vi "DimostratoreCalibrazioni-backup.vi"() -> ()   [LabVIEW 2019]
uses:
  TypeDef/SlugExpiration.ctl
  ByteGSAPIBase.lvclass
  TypeDef/CalibrationStates.ctl
  FetchCalibration/Converted_Slug_Cluster.ctl
  Instruments/Instruments.ctl
  CalibrationMeasurements/BodyCalibrazioneMisure.ctl
  aa47c742-c095-4670-bf1f-6b28e4309cef.vi
  <vilib>/numeric/Random Number (Range) I64.vi
  <vilib>/Array/Sort 2D Array - Pop Stack.vi
  <vilib>/Array/Sort 2D Array - Push Stack.vi
  <vilib>/numeric/sub_Random U32.vi
panel:
  out "Stato":string
  out "Misurazioni n.":string
  in  "Cancel":bool
  in  "Approvation":bool
  out "Tot Misurazioni":i32
  in  "Avanti":bool
  in  "Repeat":bool
  out "Esito":string
  out "Valore misurato":dbl
  out "Valore di riferimento":dbl
  out "Waveform Chart":i64(graph)
  in  "Start Calibration":bool
  in  "Next":bool
  in  "Previus":bool
  out "Misurazioni":string
  in  "Filtro":enum16{"All", "Expired", "Not Expired"}(ring)
  in  "Slug list":T1[](array[typedef])
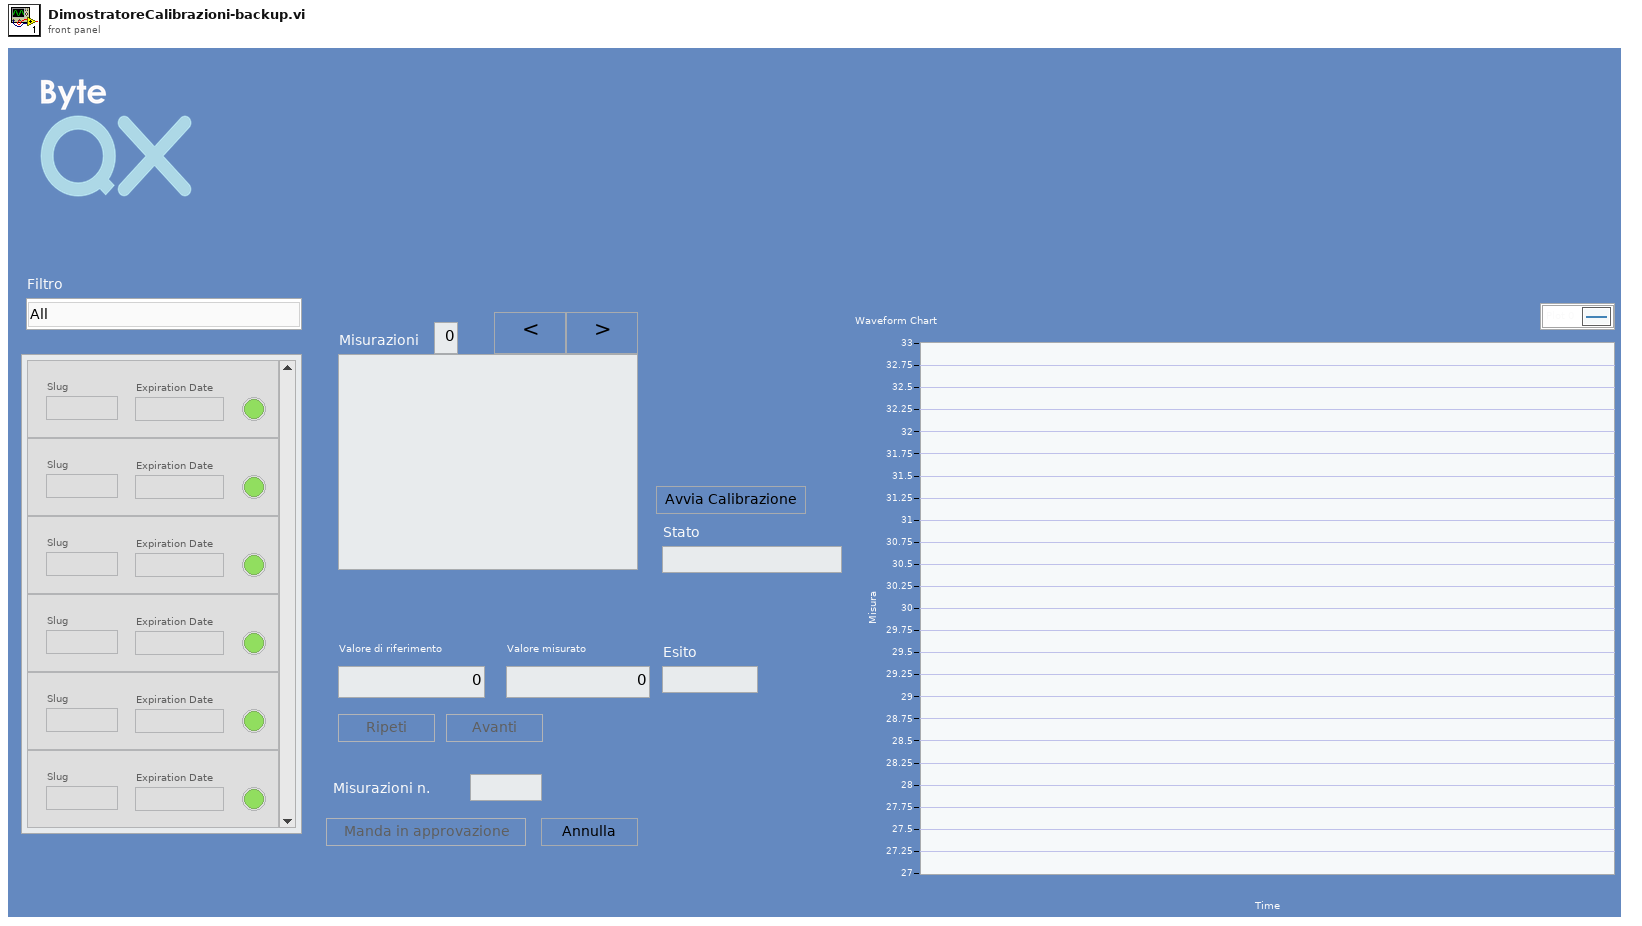
[diagram p1: front panel]
types:
  T1 = typedef "SlugExpiration.ctl" = cluster{"Slug":string, "Expiration Date":string, "Color Box":u32, "Active":bool, "Expired?":bool, "Id":i32}
  T2 = typedef "CalibrationStates.ctl" = enum16{"Init", "Idle", "GetInstruments", "Fetch", "GetCalibrations", "CheckTotalMisurations", "StartCalibration", "ManageCalibration", "Approve"}
  T3 = typedef "ByteGSWebAPI.lvlib/ByteGSAPIBase.lvclass/BodyCalibrazioneMisure.ctl" = cluster{"controls":cluster{"id":u16, "descrizione":string, "numero_misure_necessarie":u16, "riferimento_obiettivo":dbl, "mpe_max":dbl, "mpe_min":dbl, "deviazione_standard":dbl, "incertezza":dbl, "numero_misure_effettuate":u32, "temperatura_c":dbl, "umidita":dbl, "strumento_riferimento":cluster{"id":u16, "nome":string}[]}[]}
  T4 = typedef "Instruments.ctl" = cluster{"id":i32, "slug":string, "stabilimento":cluster{"id":dbl}, "categoria":cluster{"id":dbl}, "tipologia_di_visualizzazione":cluster{"id":dbl}, "stato":cluster{"id":dbl}, "descrizione":string, "costruttore":string, "matricola":string, "data_registrazione":string, "intervallo_di_taratura_mesi":dbl, "reparto":string, "campo_misura":string, "risoluzione":dbl, "responsabile_strumento":string, "classe_di_precisione":string, "classificazione":string, "appunti":string, "manuale":string, "foto":string, "riferimento":bool, "qr_hashcode":string, "costo_euro":dbl}
  T5 = typedef "ByteGSWebAPI.lvlib/ByteGSAPIBase.lvclass/Converted_Slug_Cluster.ctl" = cluster{"id":u32, "instrument":string, "name":string, "date":timestamp}
  T6 = cluster{"Esito":refnum<vi>, "Avanti":refnum<vi>, "Repeat":refnum<vi>, "Slug list":refnum<vi>, "Start Calibration":refnum<vi>, "Avanti":refnum<vi>, "Cancel":refnum<vi>, "Approvation":refnum<vi>}
  T7 = cluster{"ByteGSAPIBase in":refnum<class "ByteGSAPIBase.lvclass">, "Instruments_Slug":string[], "All_Instruments_Cals":T5[], "All_Instruments":T4[], "Slug list All":T1[], "Calibrations":T3, "Selected Slug":i32, "Misurazioni":string, "Misurazioni index":i32, "Next State":T2, "Waveform Chart":refnum<vi>, "New Val":dbl, "Id Failed":u32, "Failed?":bool, "Cal Index":i32, "Misurazioni n":string, "Stato":string, "Esito":string}
  T8 = cluster{"id":u16, "descrizione":string, "numero_misure_necessarie":u16, "riferimento_obiettivo":dbl, "mpe_max":dbl, "mpe_min":dbl, "deviazione_standard":dbl, "incertezza":dbl, "numero_misure_effettuate":u32, "temperatura_c":dbl, "umidita":dbl, "strumento_riferimento":cluster{"id":u16, "nome":string}[]}[]
  T9 = cluster{"id":u16, "descrizione":string, "numero_misure_necessarie":u16, "riferimento_obiettivo":dbl, "mpe_max":dbl, "mpe_min":dbl, "deviazione_standard":dbl, "incertezza":dbl, "numero_misure_effettuate":u32, "temperatura_c":dbl, "umidita":dbl, "strumento_riferimento":cluster{"id":u16, "nome":string}[]}
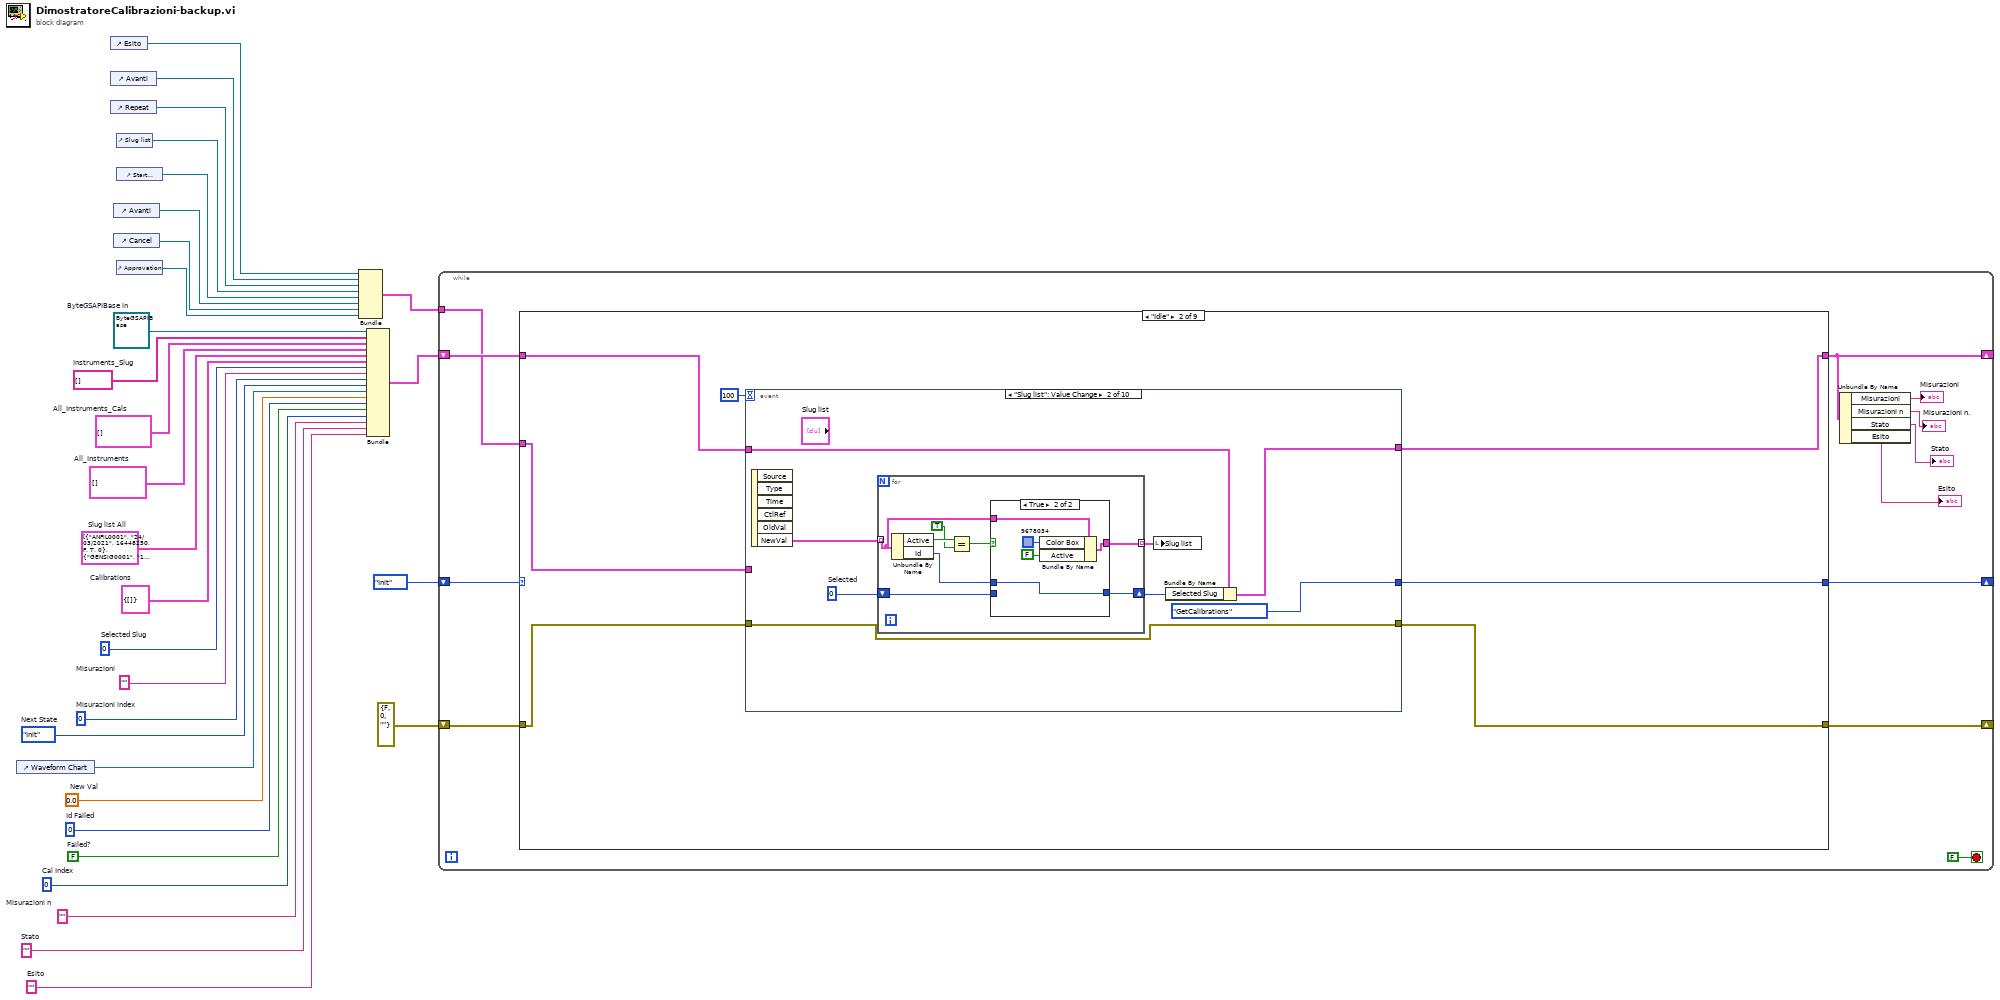
[diagram p0: block diagram]
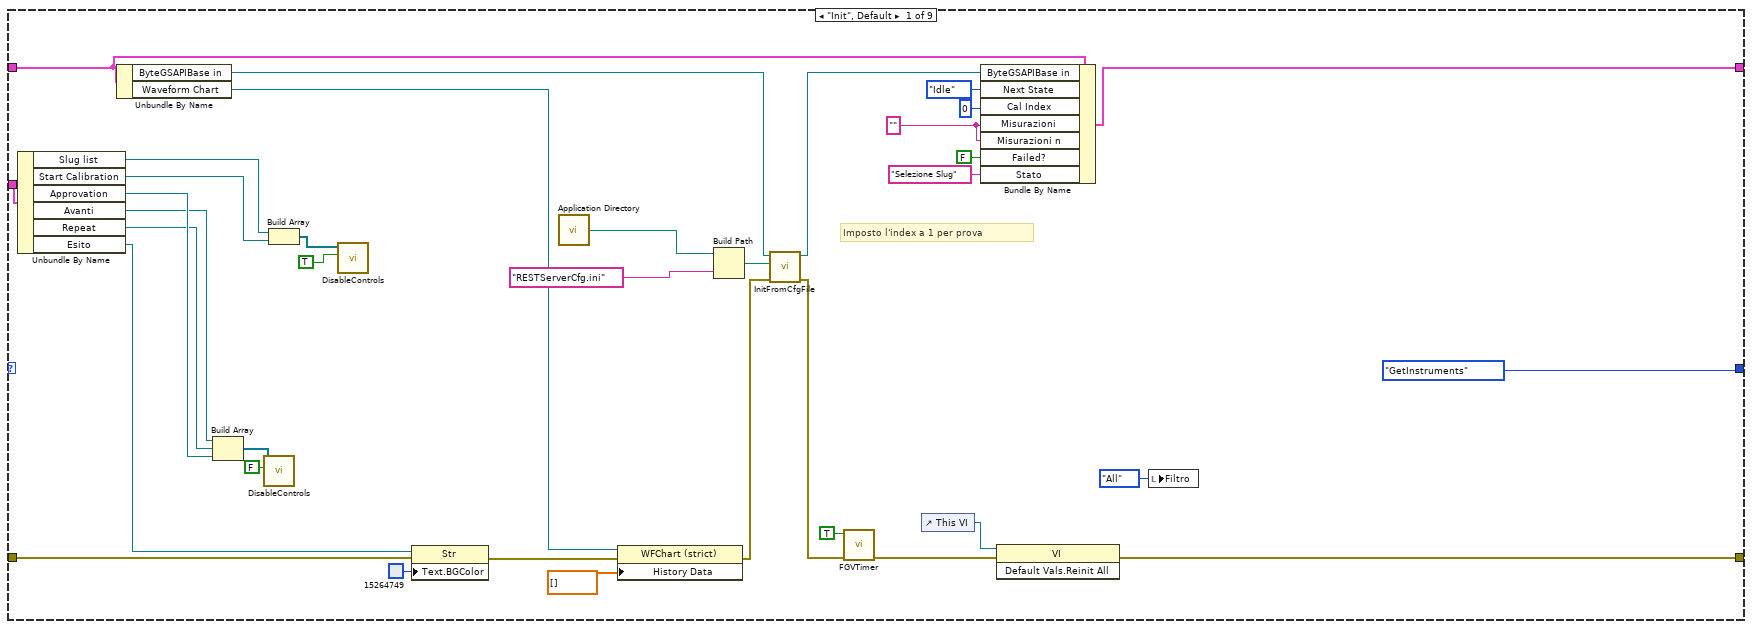
[diagram p2: hidden frame]
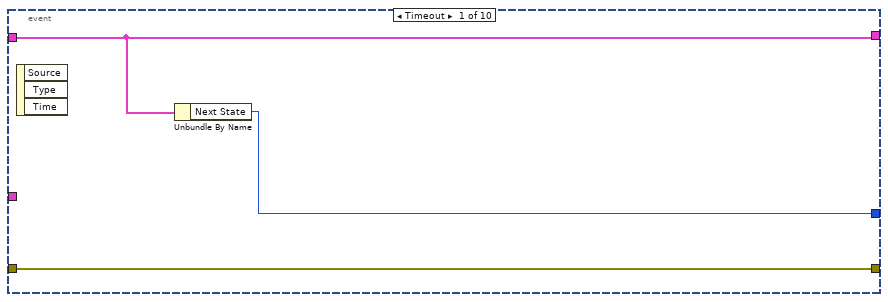
[diagram p3: hidden frame]
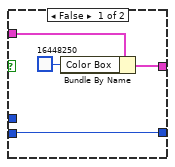
[diagram p4: hidden frame]
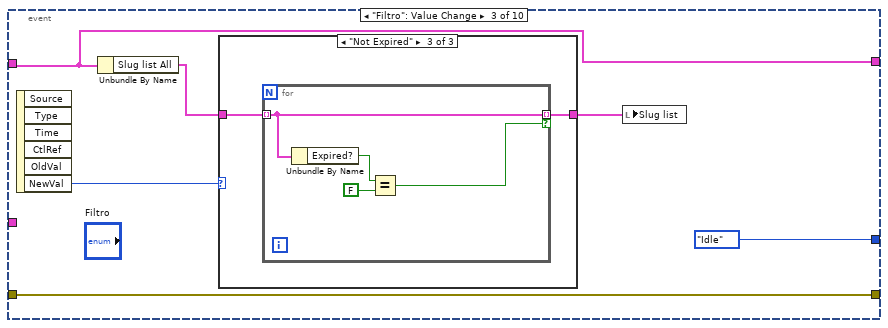
[diagram p5: hidden frame]
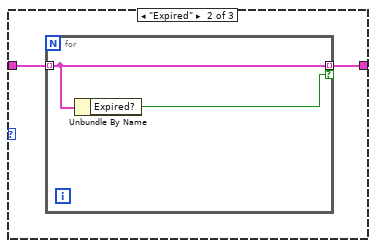
[diagram p7: hidden frame]
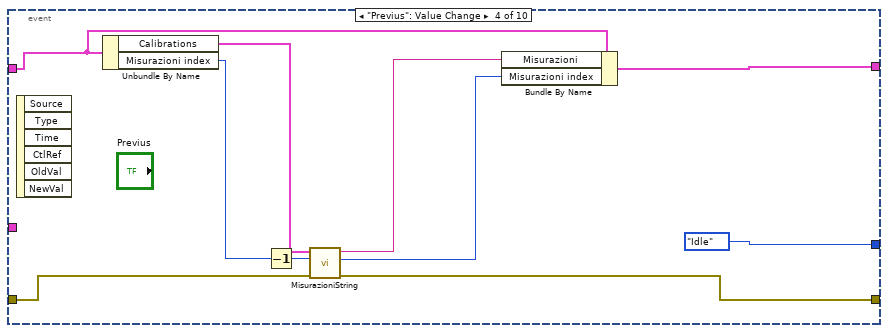
[diagram p8: hidden frame]
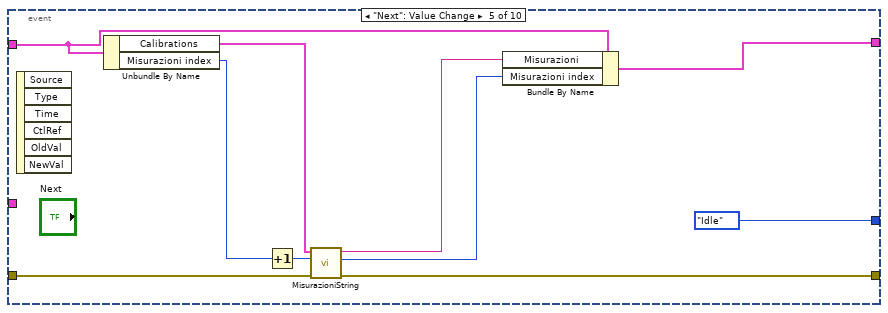
[diagram p9: hidden frame]
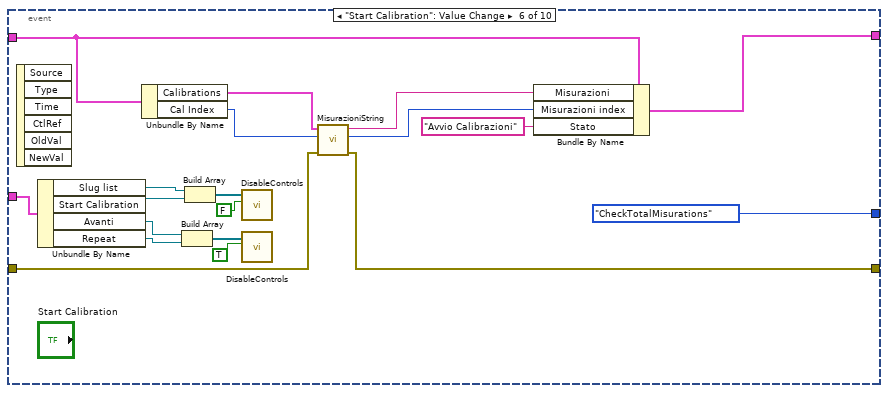
[diagram p10: hidden frame]
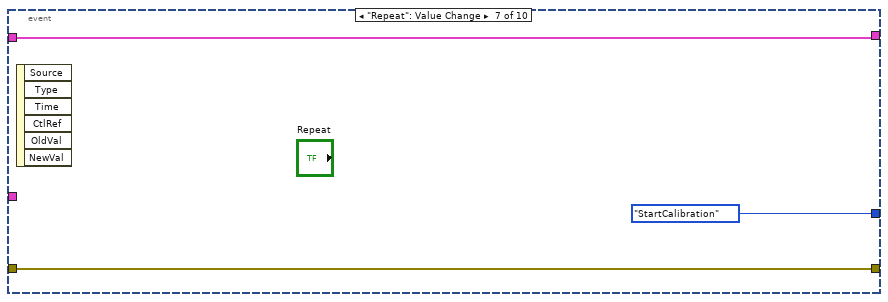
[diagram p11: hidden frame]
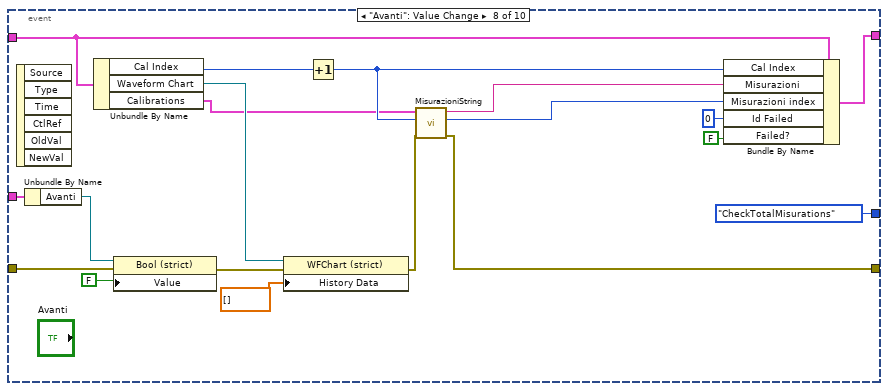
[diagram p12: hidden frame]
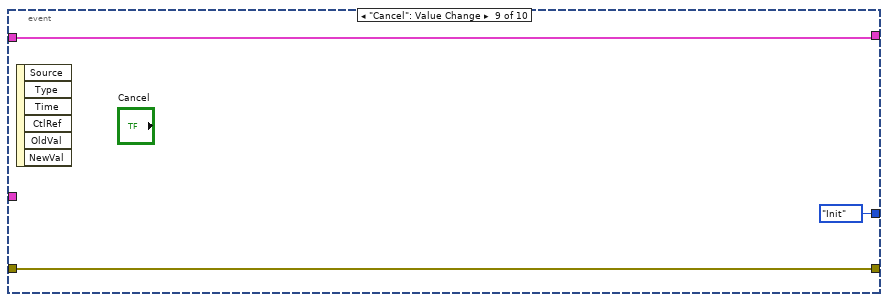
[diagram p13: hidden frame]
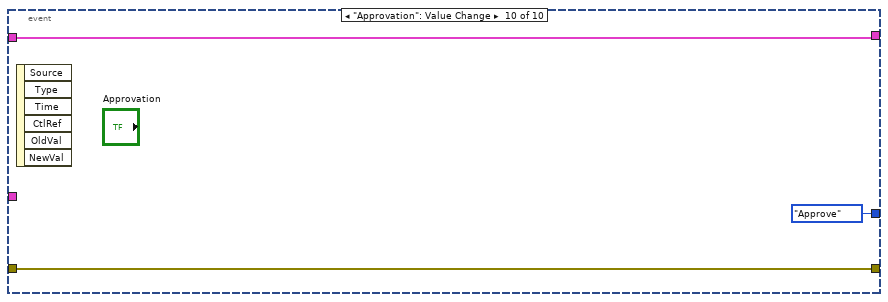
[diagram p14: hidden frame]
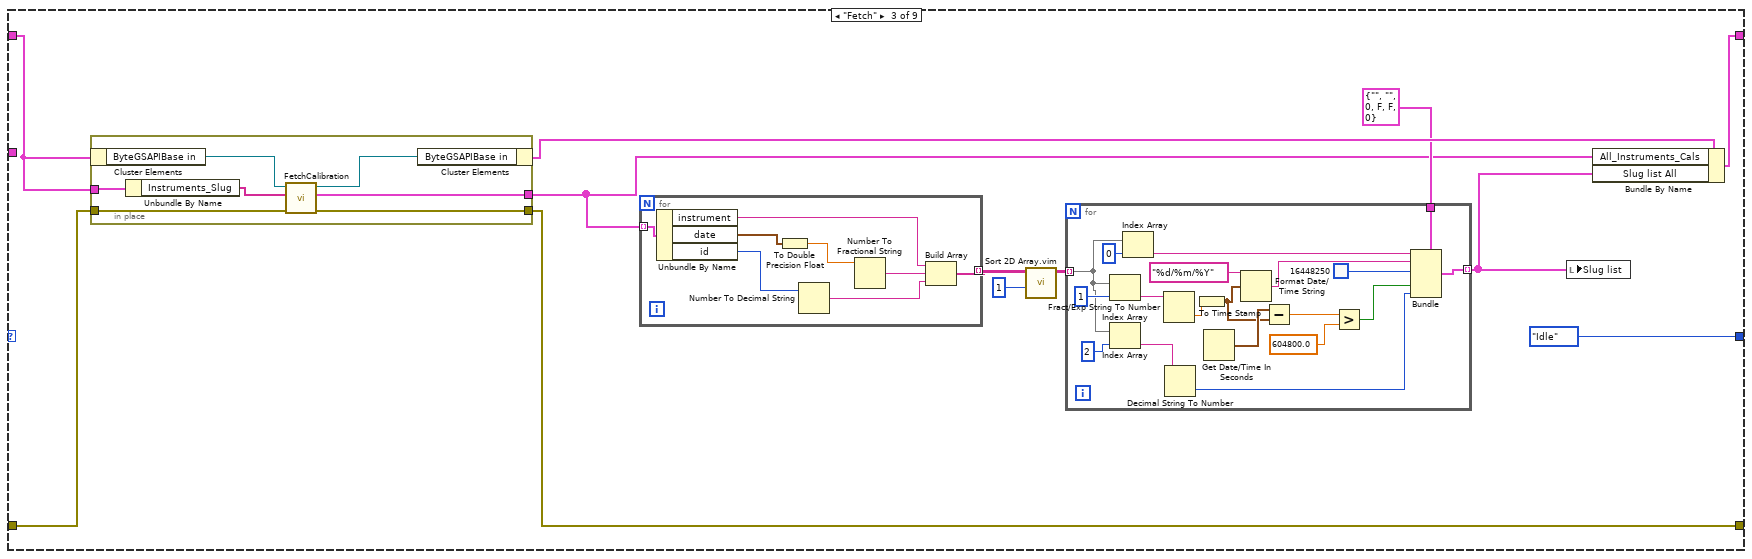
[diagram p15: hidden frame]
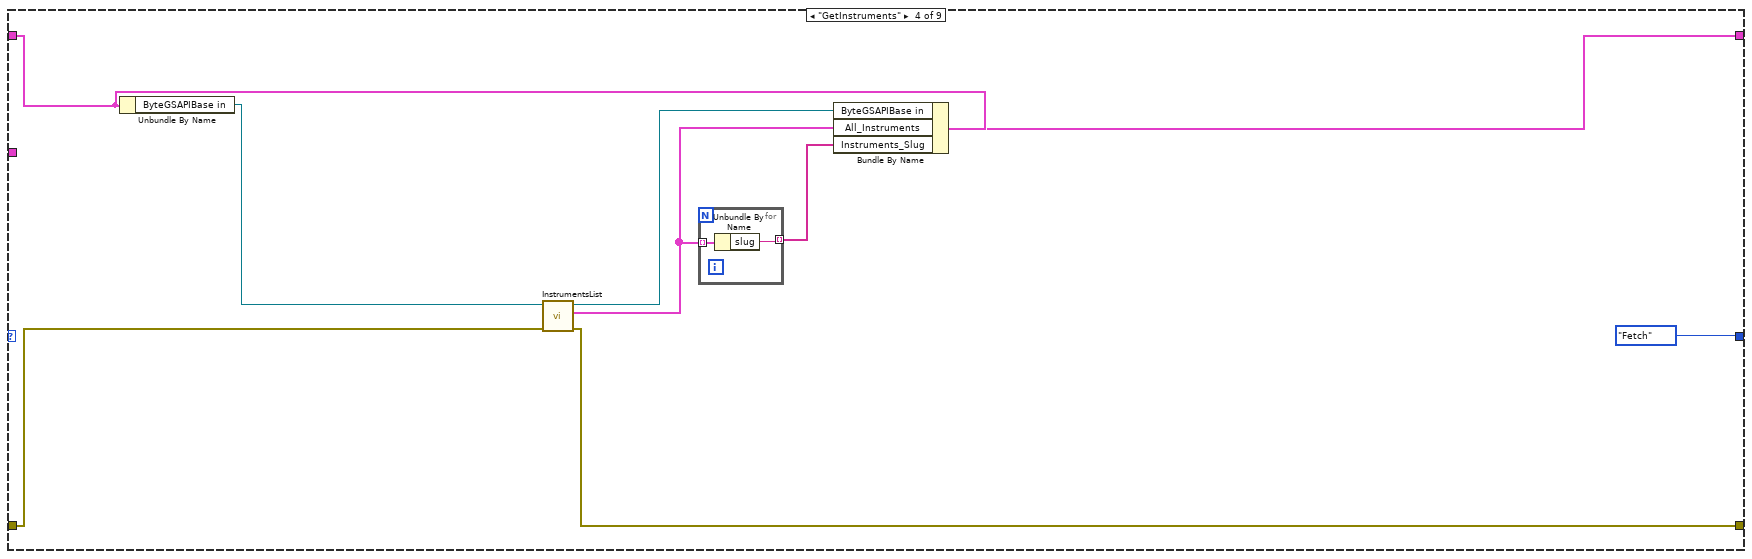
[diagram p16: hidden frame]
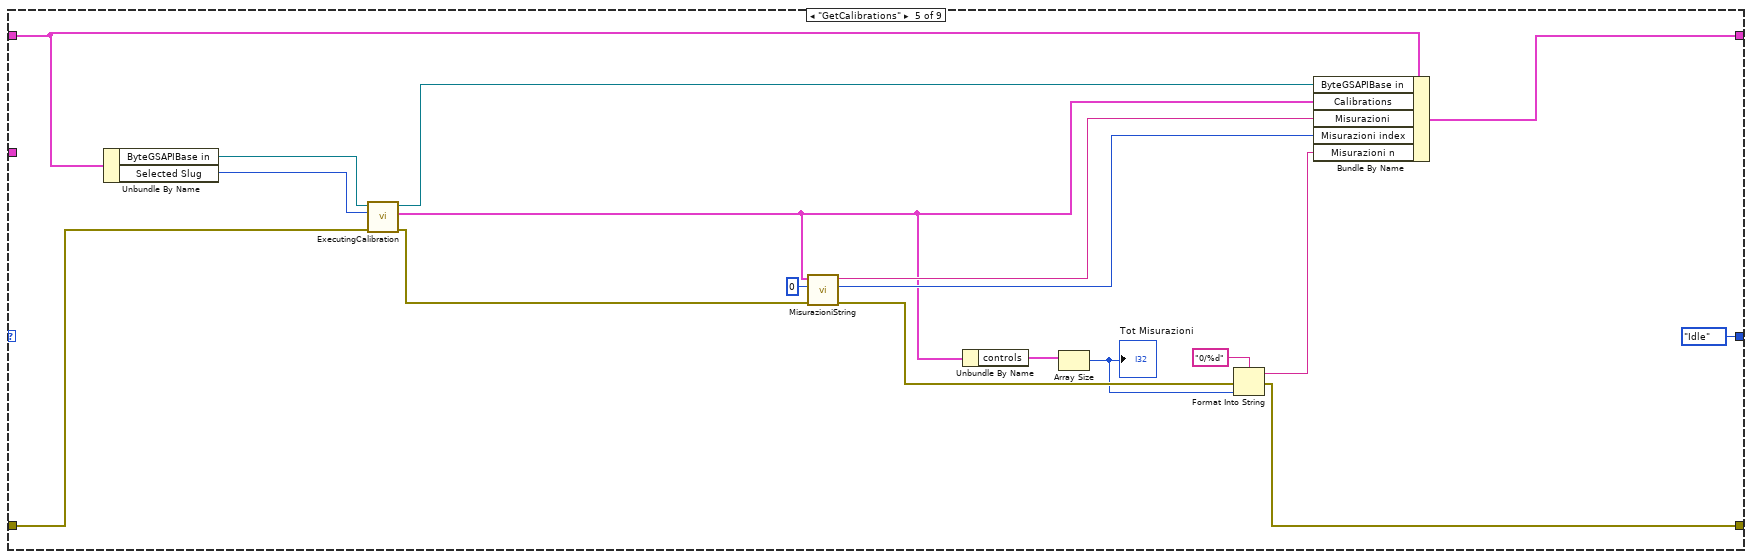
[diagram p17: hidden frame]
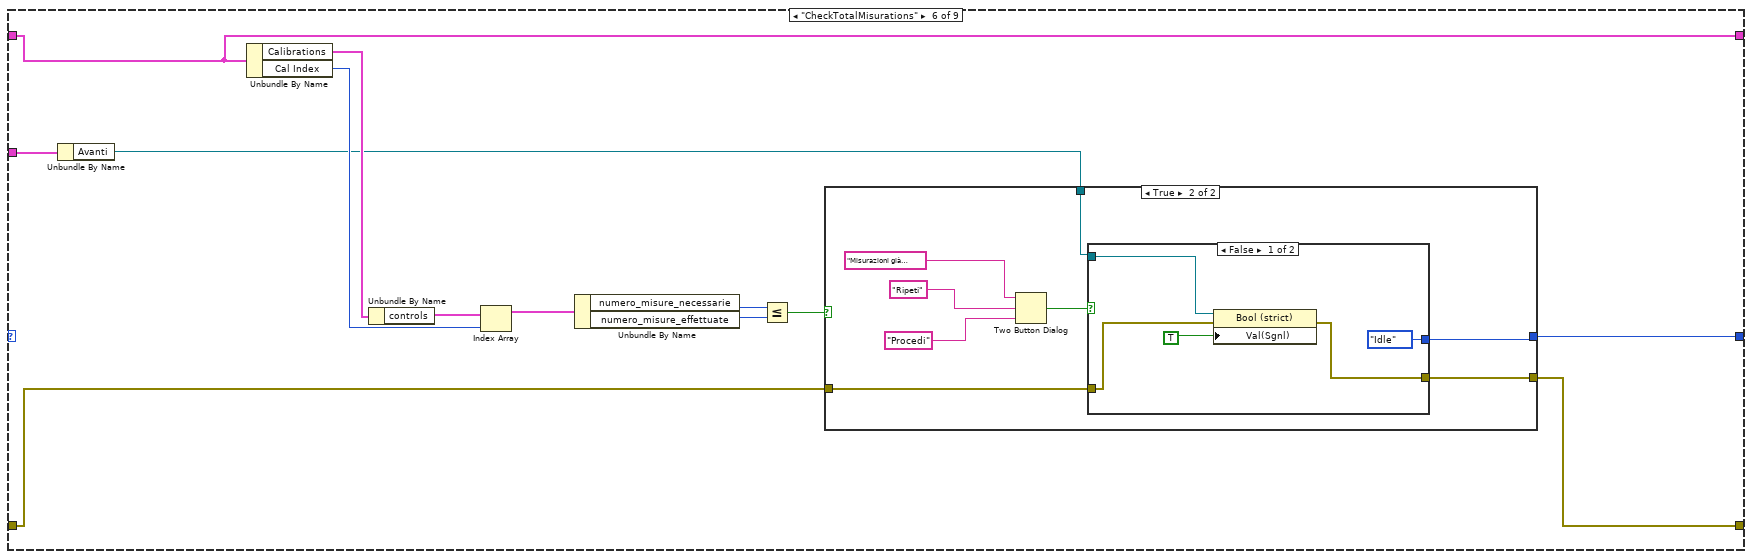
[diagram p18: hidden frame]
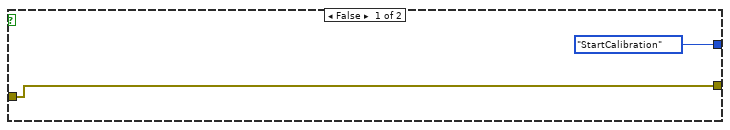
[diagram p19: hidden frame]
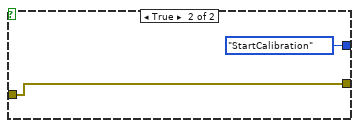
[diagram p20: hidden frame]
diagram:
  w2 = ""  # Esito
  w3 = ""  # Stato
  w8 = ""  # Misurazioni n
  w13 = 0  # Cal Index
  w14 = FALSE  # Failed?
  w15 = u32 0  # Id Failed
  w16 = 0.0  # New Val
  w18 = CalibrationStates."Init"  # Next State
  w19 = 0  # Misurazioni index
  w20 = ""  # Misurazioni
  w21 = T1[] [{"Slug"="ANFIL0001", "Expiration Date"="24/03/2021", "Color Box"=16448250, "Active"=FALSE, "Expired?"=TRUE, "Id"=0}, {"Slug"="GENSIG0001", "Expiration Date"="18/05/2021", "Color Box"=16448250, "Active"=FALSE, "Expired?"=TRUE, "Id"=0}, {"Slug"="GENSIG0001", "Expiration Date"="15/09/2021", "Color Box"=16448250, "Active"=FALSE, "Expired?"=TRUE, "Id"=0}, {"Slug"="DIN0001", "Expiration Date"="11/10/2021", "Color Box"=13816530, "Active"=FALSE, "Expired?"=TRUE, "Id"=0}, {"Slug"="DMM0002", "Expiration Date"="20/10/2021", "Color Box"=16448250, "Active"=FALSE, "Expired?"=TRUE, "Id"=0}, {"Slug"="COMP0001", "Expiration Date"="01/12/2021", "Color Box"=16448250, "Active"=FALSE, "Expired?"=TRUE, "Id"=0}, {"Slug"="TORS0002", "Expiration Date"="06/12/2021", "Color Box"=16448250, "Active"=FALSE, "Expired?"=TRUE, "Id"=0}, {"Slug"="CDIND0001", "Expiration Date"="04/03/2022", "Color Box"=16448250, "Active"=FALSE, "Expired?"=TRUE, "Id"=0}, {"Slug"="CALI0004", "Expiration Date"="11/03/2022", "Color Box"=16448250, "Active"=FALSE, "Expired?"=TRUE, "Id"=0}, {"Slug"="CALI0001", "Expiration Date"="10/05/2022", "Color Box"=16448250, "Active"=FALSE, "Expired?"=TRUE, "Id"=0}, {"Slug"="CALI0012", "Expiration Date"="10/05/2022", "Color Box"=16448250, "Active"=FALSE, "Expired?"=TRUE, "Id"=0}, {"Slug"="CALI0011", "Expiration Date"="11/05/2022", "Color Box"=16448250, "Active"=FALSE, "Expired?"=TRUE, "Id"=0}, {"Slug"="CALI0014", "Expiration Date"="04/07/2022", "Color Box"=16448250, "Active"=FALSE, "Expired?"=TRUE, "Id"=0}, {"Slug"="CDIND0001", "Expiration Date"="15/07/2022", "Color Box"=16448250, "Active"=FALSE, "Expired?"=TRUE, "Id"=0}, {"Slug"="CALI0024", "Expiration Date"="11/07/2023", "Color Box"=16448250, "Active"=FALSE, "Expired?"=TRUE, "Id"=0}, {"Slug"="CALI0017", "Expiration Date"="19/09/2023", "Color Box"=16448250, "Active"=FALSE, "Expired?"=TRUE, "Id"=0}, {"Slug"="CALI0020", "Expiration Date"="02/11/2023", "Color Box"=16448250, "Active"=FALSE, "Expired?"=TRUE, "Id"=0}, {"Slug"="CALI0017", "Expiration Date"="03/11/2023", "Color Box"=16448250, "Active"=FALSE, "Expired?"=TRUE, "Id"=0}, {"Slug"="CALI0025", "Expiration Date"="11/11/2023", "Color Box"=16448250, "Active"=FALSE, "Expired?"=TRUE, "Id"=0}, {"Slug"="CLBR0001", "Expiration Date"="30/11/2023", "Color Box"=16448250, "Active"=FALSE, "Expired?"=TRUE, "Id"=0}, {"Slug"="CLBR0001", "Expiration Date"="02/01/2024", "Color Box"=16448250, "Active"=FALSE, "Expired?"=TRUE, "Id"=0}, {"Slug"="CLBR0001", "Expiration Date"="02/01/2024", "Color Box"=16448250, "Active"=FALSE, "Expired?"=TRUE, "Id"=0}, {"Slug"="CLBR0003", "Expiration Date"="04/03/2024", "Color Box"=16448250, "Active"=FALSE, "Expired?"=TRUE, "Id"=0}, {"Slug"="MICP0001", "Expiration Date"="19/03/2024", "Color Box"=16448250, "Active"=FALSE, "Expired?"=TRUE, "Id"=0}, {"Slug"="TERM0002", "Expiration Date"="04/07/2024", "Color Box"=16448250, "Active"=FALSE, "Expired?"=TRUE, "Id"=0}, {"Slug"="ACCEL0008", "Expiration Date"="04/07/2024", "Color Box"=16448250, "Active"=FALSE, "Expired?"=TRUE, "Id"=0}, {"Slug"="ACCEL0008", "Expiration Date"="05/07/2024", "Color Box"=16448250, "Active"=FALSE, "Expired?"=TRUE, "Id"=0}, {"Slug"="ACCEL0008", "Expiration Date"="19/08/2024", "Color Box"=16448250, "Active"=FALSE, "Expired?"=TRUE, "Id"=0}, {"Slug"="TERM0002", "Expiration Date"="15/10/2024", "Color Box"=16448250, "Active"=FALSE, "Expired?"=TRUE, "Id"=0}, {"Slug"="BILA0001", "Expiration Date"="15/10/2024", "Color Box"=16448250, "Active"=FALSE, "Expired?"=TRUE, "Id"=0}, {"Slug"="CLBR0001", "Expiration Date"="15/10/2024", "Color Box"=16448250, "Active"=FALSE, "Expired?"=TRUE, "Id"=0}, {"Slug"="ACCEL0002", "Expiration Date"="15/10/2024", "Color Box"=16448250, "Active"=FALSE, "Expired?"=TRUE, "Id"=0}]  # Slug list All
  w22 = 0  # Selected Slug
  w23 = T3 {"controls"=[]}  # Calibrations
  w24 = T4[] []  # All_Instruments
  w25 = T5[] []  # All_Instruments_Cals
  w26 = string[] []  # Instruments_Slug
  w29 = refnum<class "ByteGSAPIBase.lvclass"> refnum  # ByteGSAPIBase in
  n1 = control-ref of="Waveform Chart"() -> (w17:refnum<vi>)
  n2 = control-ref of="Avanti"() -> (w4:refnum<vi>)
  n3 = control-ref of="Repeat"() -> (w5:refnum<vi>)
  n4 = control-ref of="Esito"() -> (w1:refnum<vi>)
  n5 = control-ref of="Avanti"() -> (w9:refnum<vi>)
  n6 = control-ref of="Cancel"() -> (w10:refnum<vi>)
  n7 = control-ref of="Start Calibration"() -> (w7:refnum<vi>)
  n8 = control-ref of="Approvation"() -> (w11:refnum<vi>)
  n9 = control-ref of="Slug list"() -> (w6:refnum<vi>)
  n10 = Bundle("Esito"=w1, "Avanti"=w4, "Repeat"=w5, "Slug list"=w6, "Start Calibration"=w7, "Avanti"=w9, "Cancel"=w10, "Approvation"=w11) -> (w12:T6)  [unwired: 1 in]
  n11 = Bundle("ByteGSAPIBase in"=w29, "Instruments_Slug"=w26, "All_Instruments_Cals"=w25, "All_Instruments"=w24, "Slug list All"=w21, "Calibrations"=w23, "Selected Slug"=w22, "Misurazioni"=w20, "Misurazioni index"=w19, "Next State"=w18, "Waveform Chart"=w17, "New Val"=w16, "Id Failed"=w15, "Failed?"=w14, "Cal Index"=w13, "Misurazioni n"=w8, "Stato"=w3, "Esito"=w2) -> (w28:T7)  [unwired: 1 in]
  n12 = while {
    shift-right: [w40] -> _
    shift-left: CalibrationStates."Init" -> [w41]
    shift-right: [w36] -> _
    shift-left: w28 -> [w39]
    shift-right: [w37] -> _
    shift-left: errorcluster {"status"=FALSE, "code"=0, "source"=""} ("error in (no error)") -> [w38]
    tunnel: w12 -> [w34]
    stop <- FALSE stop-if-true
    n13 = case shown="\"Idle\"" w41 {
      tunnel: [CalibrationStates."GetInstruments" w83 CalibrationStates."Idle" CalibrationStates."Fetch" CalibrationStates."Idle" w278 CalibrationStates."Idle" CalibrationStates."Idle" CalibrationStates."Idle"] -> w40
      tunnel: w39 -> [w74 w85 w209 w250 w268 w273 w323 w362 w434]
      tunnel: w38 -> [w44 w82 w208 w252 w269 w275 w303 w348 w433]
      tunnel: [w60 w81 w199 w246 w258 w274 w315 w339 w431] -> w37
      tunnel: [w72 w84 w205 w248 w267 w273 w322 w361 w425] -> w36
      tunnel: w34 -> [w62 w79 _ _ _ w277 w307 w349 w430]
      frame "Init", Default {
        w58 = "" ("Misurazioni")
        # "Imposto l'index a 1 per prova"
        n14 = Unbundle By Name(w62) -> ("Slug list"=w56:refnum<vi>, "Start Calibration"=w55:refnum<vi>, "Approvation"=w57:refnum<vi>, "Avanti"=w50:refnum<vi>, "Repeat"=w49:refnum<vi>, "Esito"=w43:refnum<vi>)
        n15 = Unbundle By Name(w74) -> ("ByteGSAPIBase in"=w75:refnum<class "ByteGSAPIBase.lvclass">, "Waveform Chart"=w66:refnum<vi>)
        n16 = Build Array(w50, w49, w57) -> (w52:refnum<vi>[])
        n17 = call "DisableControls.vi"("Visible"=FALSE, "Controls"=w52) -> ()  [unwired: 9 in, 1 out]
        n18 = Build Array(w56, w55) -> (w54:refnum<vi>[])
        n19 = call "DisableControls.vi"("Visible"=TRUE, "Controls"=w54) -> ()  [unwired: 9 in, 1 out]
        n20 = property class="Str"(reference=w43, error in=w44, "Text.BGColor"=u32 15264749 ("Text.Text Colors:BG Color")) -> (error out=w45:errorcluster)  [unwired: 1 out]
        n21 = call <vilib>:"Application Directory.vi"() -> ("Application Directory"=w76:path)
        n22 = property class="WFChart (strict)"(reference=w66, error in=w45, "History Data"=dbl[] []) -> (error out=w65:errorcluster)  [unwired: 1 out]
        n23 = Build Path(base path=w76, name or relative path="RESTServerCfg.ini") -> (appended path=w71:path)
        n24 = call-dynamic "InitFromCfgFile.vi"("error in (no error)"=w65, "configuration file path"=w71, "ByteGSAPIBase in"=w75) -> ("error out"=w69:errorcluster, "ByteGSAPIBase out"=w73:refnum<class "ByteGSAPIBase.lvclass">)  [unwired: 7 in]
        n25 = call "FGVTimer.vi"("error in"=w69, "Reset"=TRUE) -> ("error out"=w61:errorcluster)  [unwired: 7 in, 2 out]
        n26 = control-ref of="This VI"() -> (w59:refnum<vi>)
        n27 = Bundle By Name(cluster=w74, "ByteGSAPIBase in"=w73, "Next State"=CalibrationStates."Idle", "Cal Index"=0, "Misurazioni"=w58, "Misurazioni n"=w58, "Failed?"=FALSE, "Stato"="Selezione Slug") -> (w72:T7)
        n28 = invoke class="VI" method="Default Vals.Reinit All"(reference=w59, error in=w61) -> (error out=w60:errorcluster)  [unwired: 1 in, 2 out]
        n29 = local write "Filtro"(enum16{"All", "Expired", "Not Expired"}."All" ("Filter")) -> ()
      }
      frame "Idle" {
        n30 = event shown="[1] \"Slug list\": Value Change" {
          selector: _ -> [_ _ _ _ _ _ _ _ _ _]
          dyn-events: _ -> [_ _ _ _ _ _ _ _ _ _]
          timeout: 100 -> [_ _ _ _ _ _ _ _ _ _]
          tunnel: w85 -> [w87 w93 w116 w135 w145 w166 w172 w189 w192 w195]
          tunnel: [w87 w91 w116 w134 w142 w163 w172 w190 w192 w195] -> w84
          tunnel: [w86 CalibrationStates."GetCalibrations" CalibrationStates."Idle" CalibrationStates."Idle" CalibrationStates."Idle" CalibrationStates."CheckTotalMisurations" CalibrationStates."StartCalibration" CalibrationStates."CheckTotalMisurations" CalibrationStates."Init" CalibrationStates."Approve"] -> w83
          tunnel: w82 -> [w88 w89 w114 w132 w150 w162 w170 w175 w194 w197]
          tunnel: [w88 w89 w114 w131 w149 w160 w170 w182 w194 w197] -> w81
          tunnel: w79 -> [_ _ _ _ _ w161 _ w177 _ _]
          event Timeout {
            n31 = event-data() -> ()  [unwired: 1 in, 3 out]
            n32 = Unbundle By Name(w87) -> ("Next State"=w86:T2)
          }
          event "Slug list": Value Change {
            w94 = 0  # Selected
            n33 = event-data() -> ("NewVal"=w96:T1[])  [unwired: 1 in, 5 out]
            n34 = for {
              tunnel: w96 -> [w101] mode=indexing
              tunnel: [w100] -> w95 mode=indexing
              shift-right: [w98] -> w92
              shift-left: w94 -> [w99]
              n35 = Unbundle By Name(w101) -> ("Active"=w104:bool, "Id"=w97:i32)
              n36 = Equal?(x=w104, y=TRUE) -> (x = y?=w102:bool)
              n37 = case shown="True" w102 {
                tunnel: w101 -> [w107 w113]
                tunnel: [w108 w111] -> w100
                tunnel: w99 -> [w105 _]
                tunnel: [w105 w109] -> w98
                tunnel: w97 -> [_ w109]
                frame False {
                  n38 = Bundle By Name(cluster=w107, "Color Box"=u32 16448250) -> (w108:T1)
                }
                frame True {
                  n39 = Bundle By Name(cluster=w113, "Color Box"=u32 9678034, "Active"=FALSE) -> (w111:T1)
                }
              }
            }
            n40 = local write "Slug list"(w95) -> ()
            n41 = Bundle By Name(cluster=w93, "Selected Slug"=w92) -> (w91:T7)
          }
          event "Filtro": Value Change {
            n42 = event-data() -> ("NewVal"=w119:enum16{"All", "Expired", "Not Expired"})  [unwired: 1 in, 5 out]
            n43 = Unbundle By Name(w116) -> ("Slug list All"=w118:T1[])
            n44 = case shown="\"Not Expired\"" w119 {
              tunnel: w118 -> [w120 w122 w126]
              tunnel: [w120 w121 w125] -> w117
              frame "All" {
              }
              frame "Expired" {
                n45 = for {
                  tunnel: w122 -> [w124] mode=indexing
                  tunnel: [w124] -> w121 mode=indexing if=w123
                  n46 = Unbundle By Name(w124) -> ("Expired?"=w123:bool)
                }
              }
              frame "Not Expired" {
                n47 = for {
                  tunnel: w126 -> [w130] mode=indexing
                  tunnel: [w130] -> w125 mode=indexing if=w127
                  n48 = Unbundle By Name(w130) -> ("Expired?"=w129:bool)
                  n49 = Equal?(x=w129, y=FALSE) -> (x = y?=w127:bool)
                }
              }
            }
            n50 = local write "Slug list"(w117) -> ()
          }
          event "Previus": Value Change {
            n51 = event-data() -> ()  [unwired: 1 in, 6 out]
            n52 = Unbundle By Name(w135) -> ("Calibrations"=w140:T3, "Misurazioni index"=w138:i32)
            n53 = Decrement(x=w138) -> (x-1=w139:i32)
            n54 = call "MisurazioniString.vi"("error in (no error)"=w132, "index"=w139, "Calibration data"=w140) -> ("error out"=w131:errorcluster, "index"=w136:i32, "String"=w137:string)  [unwired: 6 in]
            n55 = Bundle By Name(cluster=w135, "Misurazioni"=w137, "Misurazioni index"=w136) -> (w134:T7)
          }
          event "Next": Value Change {
            n56 = event-data() -> ()  [unwired: 1 in, 6 out]
            n57 = Unbundle By Name(w145) -> ("Calibrations"=w148:T3, "Misurazioni index"=w146:i32)
            n58 = Increment(x=w146) -> (x+1=w147:i32)
            n59 = call "MisurazioniString.vi"("error in (no error)"=w150, "index"=w147, "Calibration data"=w148) -> ("error out"=w149:errorcluster, "index"=w143:i32, "String"=w144:string)  [unwired: 6 in]
            n60 = Bundle By Name(cluster=w145, "Misurazioni"=w144, "Misurazioni index"=w143) -> (w142:T7)
          }
          event "Start Calibration": Value Change {
            n61 = event-data() -> ()  [unwired: 1 in, 6 out]
            n62 = Unbundle By Name(w161) -> ("Slug list"=w159:refnum<vi>, "Start Calibration"=w158:refnum<vi>, "Avanti"=w155:refnum<vi>, "Repeat"=w154:refnum<vi>)
            n63 = Unbundle By Name(w166) -> ("Calibrations"=w168:T3, "Cal Index"=w167:i32)
            n64 = Build Array(w155, w154) -> (w153:refnum<vi>[])
            n65 = Build Array(w159, w158) -> (w157:refnum<vi>[])
            n66 = call "DisableControls.vi"("Visible"=FALSE, "Controls"=w157) -> ()  [unwired: 9 in, 1 out]
            n67 = call "DisableControls.vi"("Visible"=TRUE, "Controls"=w153) -> ()  [unwired: 9 in, 1 out]
            n68 = call "MisurazioniString.vi"("error in (no error)"=w162, "index"=w167, "Calibration data"=w168) -> ("error out"=w160:errorcluster, "index"=w164:i32, "String"=w165:string)  [unwired: 6 in]
            n69 = Bundle By Name(cluster=w166, "Misurazioni"=w165, "Misurazioni index"=w164, "Stato"="Avvio Calibrazioni") -> (w163:T7)
          }
          event "Repeat": Value Change {
            n70 = event-data() -> ()  [unwired: 1 in, 6 out]
          }
          event "Avanti": Value Change {
            n71 = event-data() -> ()  [unwired: 1 in, 6 out]
            n72 = Unbundle By Name(w177) -> ("Avanti"=w179:refnum<vi>)
            n73 = Unbundle By Name(w189) -> ("Cal Index"=w188:i32, "Waveform Chart"=w186:refnum<vi>, "Calibrations"=w184:T3)
            n74 = property class="Bool (strict)"(reference=w179, error in=w175, "Value"=FALSE) -> (error out=w176:errorcluster)  [unwired: 1 out]
            n75 = property class="WFChart (strict)"(reference=w186, error in=w176, "History Data"=dbl[] []) -> (error out=w183:errorcluster)  [unwired: 1 out]
            n76 = Increment(x=w188) -> (x+1=w185:i32)
            n77 = call "MisurazioniString.vi"("error in (no error)"=w183, "index"=w185, "Calibration data"=w184) -> ("error out"=w182:errorcluster, "index"=w180:i32, "String"=w181:string)  [unwired: 6 in]
            n78 = Bundle By Name(cluster=w189, "Cal Index"=w185, "Misurazioni"=w181, "Misurazioni index"=w180, "Id Failed"=u32 0, "Failed?"=FALSE) -> (w190:T7)
          }
          event "Cancel": Value Change {
            n79 = event-data() -> ()  [unwired: 1 in, 6 out]
          }
          event "Approvation": Value Change {
            n80 = event-data() -> ()  [unwired: 1 in, 6 out]
          }
        }
      }
      frame "Fetch" {
        n81 = in-place {
          in-place-border: w208 -> [w242]
          in-place-border: [w241] -> w199
          in-place-border: [w240] -> w198
          in-place-border: w209 -> [w238]
          n82 = in-place-cluster #1(w209) -> ("ByteGSAPIBase in"=w239:refnum<class "ByteGSAPIBase.lvclass">)
          n83 = Unbundle By Name(w238) -> ("Instruments_Slug"=w237:string[])
          n84 = call "FetchCalibration.vi"("error in (no error)"=w242, "Instruments"=w237, "ByteGSAPIBase in"=w239) -> ("error out"=w241:errorcluster, "Instruments"=w240:T5[], "ByteGSAPIBase out"=w243:refnum<class "ByteGSAPIBase.lvclass">)  [unwired: 6 in]
          n85 = in-place-cluster #1("ByteGSAPIBase in"=w243) -> (w206:T7)
        }
        n86 = for {
          tunnel: w198 -> [w236] mode=indexing
          tunnel: [w235] -> w204 mode=indexing
          n87 = Unbundle By Name(w236) -> ("instrument"=w234:string, "date"=w233:timestamp, "id"=w230:u32)
          n88 = To Double Precision Float(number=w233) -> (double precision float=w232:dbl)
          n89 = Number To Decimal String(number=w230) -> (decimal integer string=w229:string)  [unwired: 1 in]
          n90 = Number To Fractional String(number=w232) -> (F-format string=w231:string)  [unwired: 3 in]
          n91 = Build Array(w234, w231, w229) -> (w235:string[])
        }
        n92 = call "Sort 2D Array.vim"("index"=1, "2D array"=w204) -> ("sorted 2D array"=w202:string[][])  [unwired: 8 in, 1 out]
        n93 = for {
          tunnel: w202 -> [w212] mode=indexing
          tunnel: T1 {"Slug"="", "Expiration Date"="", "Color Box"=0, "Active"=FALSE, "Expired?"=FALSE, "Id"=0} ("Cluster") -> [w228]
          tunnel: [w219] -> w200 mode=indexing
          n94 = Index Array(array=w212, index=1) -> (element=w223:string)
          n95 = Index Array(array=w212, index=2) -> (element=w211:string)
          n96 = Index Array(array=w212, index=0) -> (element=w225:string)
          n97 = Fract/Exp String To Number(string=w223) -> (number=w222:dbl)  [unwired: 3 in, 1 out]
          n98 = Decimal String To Number(string=w211) -> (number=w210:i32)  [unwired: 2 in, 1 out]
          n99 = To Time Stamp(1:w222) -> (0:w214:timestamp)
          n100 = Get Date/Time In Seconds() -> (seconds since 1Jan1904=w215:timestamp)
          n101 = Format Date/Time String(time format string (%c)="%d/%m/%Y", seconds (now)=w214) -> (date/time string=w220:string)  [unwired: 1 in]
          n102 = Subtract(x=w215, y=w214) -> (x-y=w218:dbl)
          n103 = Greater?(x=w218, y=604800.0) -> (0:w216:bool)
          n104 = Bundle(cluster=w228, "Slug"=w225, "Expiration Date"=w220, "Color Box"=u32 16448250, "Expired?"=w216, "Id"=w210) -> (w219:T1)  [unwired: 1 in]
        }
        n105 = local write "Slug list"(w200) -> ()
        n106 = Bundle By Name(cluster=w206, "All_Instruments_Cals"=w198, "Slug list All"=w200) -> (w205:T7)
      }
      frame "GetInstruments" {
        n107 = Unbundle By Name(w250) -> ("ByteGSAPIBase in"=w251:refnum<class "ByteGSAPIBase.lvclass">)
        n108 = call "InstrumentsList.vi"("error in (no error)"=w252, "ByteGSAPIBase in"=w251) -> ("error out"=w246:errorcluster, "Array"=w245:T4[], "ByteGSAPIBase out"=w249:refnum<class "ByteGSAPIBase.lvclass">)  [unwired: 7 in]
        n109 = for {
          tunnel: w245 -> [w254] mode=indexing
          tunnel: [w253] -> w244 mode=indexing
          n110 = Unbundle By Name(w254) -> ("slug"=w253:string)
        }
        n111 = Bundle By Name(cluster=w250, "ByteGSAPIBase in"=w249, "All_Instruments"=w245, "Instruments_Slug"=w244) -> (w248:T7)
      }
      frame "GetCalibrations" {
        n112 = Unbundle By Name(w268) -> ("ByteGSAPIBase in"=w270:refnum<class "ByteGSAPIBase.lvclass">, "Selected Slug"=w271:i32)
        n113 = call "ExecutingCalibration.vi"("error in (no error)"=w269, "calibration_id"=w271, "ByteGSAPIBase in"=w270) -> ("error out"=w265:errorcluster, "Calibration data"=w261:T3, "ByteGSAPIBase out"=w266:refnum<class "ByteGSAPIBase.lvclass">)  [unwired: 6 in]
        n114 = call "MisurazioniString.vi"("error in (no error)"=w265, "index"=0, "Calibration data"=w261) -> ("error out"=w259:errorcluster, "index"=w262:i32, "String"=w264:string)  [unwired: 6 in]
        n115 = Unbundle By Name(w261) -> ("controls"=w260:T8)
        n116 = Array Size(array=w260) -> (size(s)=w256:i32)
        "Tot Misurazioni" <- w256
        n117 = Format Into String(format string="0/%d", error in=w259, w256) -> (resulting string=w255:string, error out=w258:errorcluster)  [unwired: 1 in]
        n118 = Bundle By Name(cluster=w268, "ByteGSAPIBase in"=w266, "Calibrations"=w261, "Misurazioni"=w264, "Misurazioni index"=w262, "Misurazioni n"=w255) -> (w267:T7)
      }
      frame "CheckTotalMisurations" {
        n119 = Unbundle By Name(w277) -> ("Avanti"=w276:refnum<vi>)
        n120 = Unbundle By Name(w273) -> ("Calibrations"=w285:T3, "Cal Index"=w282:i32)
        n121 = Unbundle By Name(w285) -> ("controls"=w284:T8)
        n122 = Index Array(array=w284, index=w282) -> (element=w283:T9)
        n123 = Unbundle By Name(w283) -> ("numero_misure_necessarie"=w281:u16, "numero_misure_effettuate"=w280:u32)
        n124 = Less Or Equal?(x=w281, y=w280) -> (x <= y?=w279:bool)
        n125 = case shown="True" w279 {
          tunnel: [CalibrationStates."StartCalibration" w291] -> w278
          tunnel: w276 -> [_ w290]
          tunnel: w275 -> [w286 w289]
          tunnel: [w286 w288] -> w274
          frame False {
          }
          frame True {
            n126 = Two Button Dialog(message="Misurazioni già completate, vuoi ripetere una misurazione o procedere con un'altra misurazione? ", 1:"Procedi" ("F button name (\"Cancel\")"), 2:"Ripeti" ("T button name (\"OK\")")) -> (T button?=w292:bool)
            n127 = case shown="False" w292 {
              tunnel: [CalibrationStates."Idle" CalibrationStates."StartCalibration"] -> w291
              tunnel: w290 -> [w299 _]
              tunnel: w289 -> [w298 w301]
              tunnel: [w297 w301] -> w288
              frame False {
                n128 = property class="Bool (strict)"(reference=w299, error in=w298, "Val(Sgnl)"=TRUE) -> (error out=w297:errorcluster)  [unwired: 1 out]
              }
              frame True {
              }
            }
          }
        }
      }
      frame "StartCalibration" {
        n129 = Unbundle By Name(w307) -> ("Esito"=w306:refnum<vi>)
        n130 = Unbundle By Name(w323) -> ("Calibrations"=w327:T3, "New Val"=w320:dbl, "Cal Index"=w314:i32)  [unwired: 1 out]
        n131 = property class="Str"(reference=w306, error in=w303, "Text.BGColor"=u32 15264749 ("Text.Text Colors:BG Color")) -> (error out=w304:errorcluster)  [unwired: 1 out]
        n132 = Unbundle By Name(w327) -> ("controls"=w311:T8)
        n133 = call "FGVTimer.vi"("error in"=w304) -> ("error out"=w316:errorcluster, "Elapsed?"=w324:bool)  [unwired: 8 in, 1 out]
        n134 = Index Array(array=w311, index=w314) -> (element=w326:T9)
        n135 = Unbundle By Name(w326) -> ("riferimento_obiettivo"=w318:dbl)
        "Valore di riferimento" <- w318
        n136 = case shown="False" w324 {
          tunnel: w318 -> [w334 _]
          tunnel: [CalibrationStates."StartCalibration" CalibrationStates."ManageCalibration"] -> w321
          tunnel: [w328 w337] -> w319
          tunnel: w320 -> [_ w337]
          frame False {
            n137 = Quotient & Remainder(x=w334, y=10.0) -> (floor(x/y)=w333:dbl)  [unwired: 1 out]
            n138 = Add(x=w334, y=w333) -> (x+y=w332:dbl)
            n139 = Subtract(x=w334, y=w333) -> (x-y=w329:dbl)
            n140 = To Quad Integer(1:w332) -> (0:w331:i64)
            n141 = To Quad Integer(1:w329) -> (0:w330:i64)
            n142 = call-poly <vilib>:"Random Number (Range).vi"("lower bound (-100)"=w330, "upper bound (100)"=w331) -> ("number"=w328:i64)  [unwired: 9 in]
            "Waveform Chart" <- w328
          }
          frame True {
          }
        }
        "Valore misurato" <- w319
        n143 = Increment(x=w314) -> (x+1=w313:i32)
        n144 = Array Size(array=w311) -> (size(s)=w312:i32)
        n145 = Format Into String(format string="%d/%d", error in=w316, w313, w312) -> (resulting string=w310:string, error out=w315:errorcluster)  [unwired: 1 in]
        n146 = Bundle By Name(cluster=w323, "Next State"=w321, "New Val"=w319, "Misurazioni n"=w310, "Stato"="Calibrazione in corso", "Esito"="...") -> (w322:T7)
      }
      frame "ManageCalibration" {
        n147 = Unbundle By Name(w362) -> ("ByteGSAPIBase in"=w365:refnum<class "ByteGSAPIBase.lvclass">, "Calibrations"=w368:T3, "New Val"=w364:dbl, "Id Failed"=w360:u32, "Failed?"=w357:bool, "Cal Index"=w351:i32)
        n148 = Unbundle By Name(w349) -> ("Approvation"=w346:refnum<vi>, "Avanti"=w345:refnum<vi>, "Esito"=w341:refnum<vi>)
        n149 = Unbundle By Name(w368) -> ("controls"=w354:T8)
        n150 = Array Size(array=w354) -> (size(s)=w353:i32)
        n151 = Decrement(x=w353) -> (x-1=w352:i32)
        n152 = Equal?(x=w352, y=w351) -> (x = y?=w350:bool)
        n153 = case shown="True" w350 {
          tunnel: w348 -> [w379 w386]
          tunnel: [w379 w386] -> w347
          tunnel: w346 -> [_ w382]
          tunnel: w345 -> [_ w385]
          frame False {
          }
          frame True {
            n154 = Build Array(w382) -> (w381:refnum<vi>[])
            n155 = Build Array(w385) -> (w384:refnum<vi>[])
            n156 = call "DisableControls.vi"("Visible"=TRUE, "Controls"=w381) -> ()  [unwired: 9 in, 1 out]
            n157 = call "DisableControls.vi"("Visible"=FALSE, "Controls"=w384) -> ()  [unwired: 9 in, 1 out]
          }
        }
        n158 = Index Array(array=w354, index=w351) -> (element=w367:T9)
        n159 = Unbundle By Name(w367) -> ("id"=w366:u16, "riferimento_obiettivo"=w363:dbl)
        n160 = disable-structure shown="Disabled" {
          disable-tunnel: w366 -> [w401 _]
          disable-tunnel: w365 -> [w400 w417]
          disable-tunnel: w364 -> [w399 w420]
          disable-tunnel: w363 -> [w398 w421]
          disable-tunnel: w347 -> [w397 w419]
          disable-tunnel: [w393 w419] -> w340
          disable-tunnel: w360 -> [w391 _]
          disable-tunnel: [w390 w417] -> w359
          disable-tunnel: [w389 _] -> w358
          disable-tunnel: w357 -> [w388 _]
          disable-tunnel: [w387 w418] -> w343
          frame Disabled {
            n161 = case shown="True" w388 {
              tunnel: w400 -> [w408 w415]
              tunnel: w398 -> [w407 _]
              tunnel: w399 -> [w406 w413]
              tunnel: w397 -> [w405 w414]
              tunnel: [w404 w411] -> w396
              tunnel: w401 -> [w402 w410]
              tunnel: [w403 w412] -> w395
              tunnel: [w402 w410] -> w394
              tunnel: w391 -> [_ w409]
              frame False {
                n162 = call-dynamic "AddMeasurement.vi"("measurement_group id"=w402, "error in (no error)"=w405, "misura_strumento"=w406, "misura_riferimento"=w407, "ByteGSAPIBase in"=w408) -> ("error out"=w404:errorcluster, "ByteGSAPIBase out"=w403:refnum<class "ByteGSAPIBase.lvclass">)  [unwired: 4 in, 1 out]
              }
              frame True {
                n163 = call-dynamic "EditMeasurement.vi"("error in (no error)"=w414, "instrument measure"=w413, "measurement id"=w409, "ByteGSAPIBase in"=w415) -> ("error out"=w411:errorcluster, "ByteGSAPIBase out"=w412:refnum<class "ByteGSAPIBase.lvclass">)  [unwired: 5 in, 1 out]
              }
            }
            n164 = call "MeasGroupResult.vi"("error in (no error)"=w396, "measurement_group_id"=w394, "ByteGSAPIBase in"=w395) -> ("error out"=w393:errorcluster, "measurements"=w392:cluster{"id":u32, "passed":bool}[], "ByteGSAPIBase out"=w390:refnum<class "ByteGSAPIBase.lvclass">)  [unwired: 5 in, 1 out]
            n165 = call "GetResult.vi"("measurements"=w392) -> ("passed"=w387:bool, "id"=w389:u32)  [unwired: 1 in]
          }
          frame Enabled {
            n166 = Equal?(x=w421, y=w420) -> (x = y?=w416:bool)
            n167 = case shown="False" w416 {
              tunnel: [TRUE FALSE] -> w418
              frame False {
              }
              frame True {
              }
            }
          }
        }
        n168 = case shown="False" w343 {
          tunnel: ["Passato" ("Esito") "Fallito" ("Esito")] -> w342
          tunnel: w341 -> [w372 w376]
          tunnel: w340 -> [w370 w375]
          tunnel: [w369 w374] -> w339
          frame False {
            n169 = property class="Str"(reference=w372, error in=w370, "Text.BGColor"=u32 6618880 ("Text.Text Colors:BG Color")) -> (error out=w369:errorcluster)  [unwired: 1 out]
          }
          frame True {
            n170 = property class="Str"(reference=w376, error in=w375, "Text.BGColor"=u32 16737380 ("Text.Text Colors:BG Color")) -> (error out=w374:errorcluster)  [unwired: 1 out]
          }
        }
        n171 = Bundle By Name(cluster=w362, "ByteGSAPIBase in"=w359, "Id Failed"=w358, "Failed?"=w343, "Next State"=CalibrationStates."Idle", "Stato"="Risultato calibrazione", "Esito"=w342) -> (w361:T7)
      }
      frame "Approve" {
        n172 = Unbundle By Name(w430) -> ("Approvation"=w429:refnum<vi>)
        n173 = Build Array(w429) -> (w428:refnum<vi>[])
        n174 = call "DisableControls.vi"("Visible"=FALSE, "Controls"=w428) -> ()  [unwired: 9 in, 1 out]
        n175 = disable-structure shown="Disabled" {
          disable-tunnel: w434 -> [w435 w446]
          disable-tunnel: w433 -> [w438 w445]
          disable-tunnel: [w437 w446] -> w426
          disable-tunnel: [w436 w445] -> w431
          frame Disabled {
            n176 = in-place {
              in-place-border: w435 -> [w442]
              in-place-border: [w441] -> w436
              in-place-border: w438 -> [w439]
              n177 = in-place-cluster #2(w435) -> ("ByteGSAPIBase in"=w444:refnum<class "ByteGSAPIBase.lvclass">)
              n178 = Unbundle By Name(w442) -> ("Selected Slug"=w440:i32)
              n179 = call "RequestApproval.vi"("error in (no error)"=w439, "calibration_id"=w440, "ByteGSAPIBase in"=w444) -> ("error out"=w441:errorcluster, "ByteGSAPIBase out"=w443:refnum<class "ByteGSAPIBase.lvclass">)  [unwired: 6 in, 1 out]
              n180 = in-place-cluster #2("ByteGSAPIBase in"=w443) -> (w437:T7)
            }
          }
          frame Enabled {
          }
        }
        n181 = Bundle By Name(cluster=w426, "Stato"="Approvazione inviata") -> (w425:T7)
      }
    }
    n182 = Unbundle By Name(w36) -> ("Misurazioni"=→"Misurazioni":string, "Misurazioni n"=→"Misurazioni n.":string, "Stato"=→"Stato":string, "Esito"=→"Esito":string)
  }
